vi "TestRegistryvi.vi"() -> ()   [LabVIEW 2012]
uses:
  <vilib>/registry/registry.llb/Registry RtKey.ctl
  <vilib>/registry/registry.llb/Read Registry Value Simple STR.vi
  <vilib>/registry/registry.llb/Registry View.ctl
panel:
  out "String/Binary data":string
  # "HKEY_LOCAL_MACHINE\\SOFTWARE\\Microsoft\\Windows\\CurrentVersion\\Installer\\UserData\\S-1-5-18\\Products\\9D764CC48C2C92E49AFCCBBFE4D2710A\\InstallProperties"
  # "HKEY_LOCAL_MACHINE\\SOFTWARE\\Microsoft\\Windows\\CurrentVersion\\Uninstall"
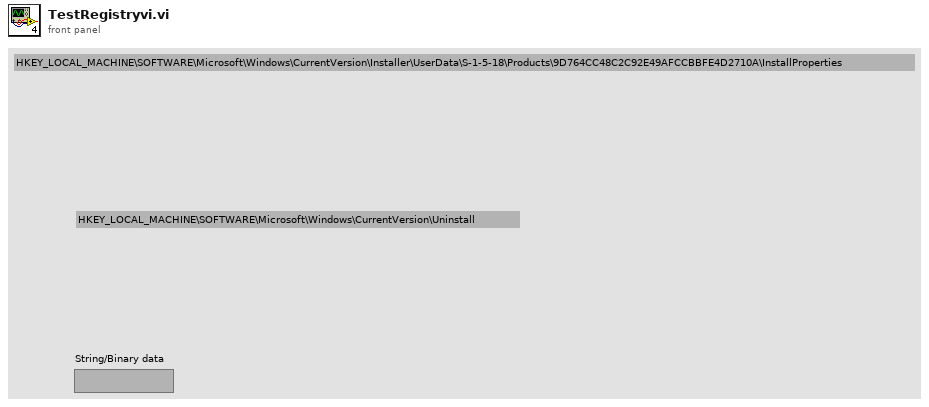
[diagram p1: front panel]
types:
  T1 = typedef "Registry View.ctl" = u16
  T2 = typedef "Registry RtKey.ctl" = enum32{"HKEY_CLASSES_ROOT", "HKEY_CURRENT_USER", "HKEY_LOCAL_MACHINE", "HKEY_USERS", "HKEY_PERFORMANCE_DATA", "HKEY_CURRENT_CONFIG", "HKEY_DYN_DATA"}
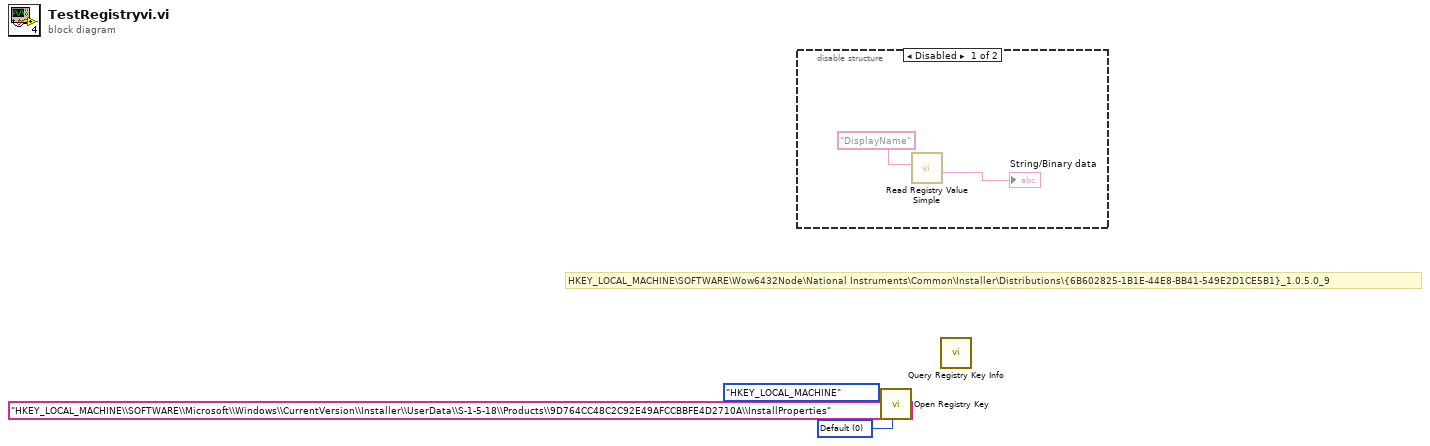
[diagram p0: block diagram]
diagram:
  w1 = T1 0 items=["Default"=0, "KEY_WOW64_64KEY"=8, "KEY_WOW64_32KEY"=9] ("registry view")
  # "HKEY_LOCAL_MACHINE\\SOFTWARE\\Wow6432Node\\National Instruments\\Common\\Installer\\Distributions\\{6B602825-1B1E-44E8-BB41-549E2D1CE5B1}_1.0.5.0_9"
  n1 = disable-structure shown="Disabled" {
    frame Disabled {
      n2 = call-poly <vilib>:"Read Registry Value Simple.vi"("value"="DisplayName") -> ("String/Binary data"=→"String/Binary data":string)  [unwired: 5 in, 3 out]
    }
    frame Enabled {
    }
  }
  n3 = call <vilib>:"Open Registry Key.vi"("registry view"=w1, "subkey"="HKEY_LOCAL_MACHINE\\SOFTWARE\\Microsoft\\Windows\\CurrentVersion\\Installer\\UserData\\S-1-5-18\\Products\\9D764CC48C2C92E49AFCCBBFE4D2710A\\InstallProperties", "root key (HKEY_LOCAL_MACHINE)"=Registry_RtKey."HKEY_LOCAL_MACHINE") -> ()  [unwired: 7 in, 2 out]
  n4 = call <vilib>:"Query Registry Key Info.vi"() -> ()  [unwired: 7 in, 5 out]
